vi "Plugin Page.vi"(8 "error in (no error)":errorcluster, 11 "Node Ptr":T1 format="%.0x") -> (0 "error out":errorcluster)   [LabVIEW 2020, in "DSF System Explorer.lvlib"]
uses:
  DSF System Explorer.lvlib
  <vilib>/NI VeriStand/Custom Device API/Custom Device Item Ref.ctl
  DSF Core.lvlibp/Classes/Component User Interface/UI Type.ctl
  <vilib>/NI VeriStand/Custom Device API/Custom Device API.lvlib
  DSF Shared.lvlib
  DSF Core.lvlibp/Classes/Component User Interface/Component User Interfaces.lvclass
  DSF Core.lvlibp/Classes/User Interface/User Interface.lvclass
panel:
  in  "Tab Control":enum32{"Settings"}(tab)
  in  "Priority":u64
  in  "Decimation":u64
  in  "Offset":u64
  in  "Header":cluster{"Section Name":string}={"Section Name"="Plugin"}
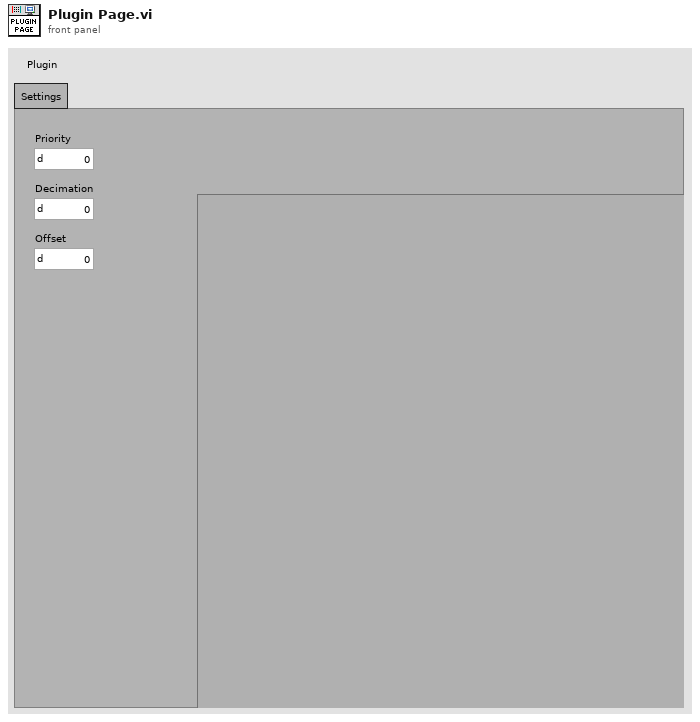
[diagram p1: front panel]
types:
  T1 = typedef "Custom Device API.lvlib/Custom Device Item Ref.ctl" = u64
  T2 = typedef "DSF Core.lvlibp/Component User Interfaces.lvclass/UI Type.ctl" = enum16{"Plugin", "Thread", "Rx Group", "Tx Group", "Rx Transfer", "Tx Transfer", "Rx Channel", "Tx Channel"}
  T3 = typedef "DSF Core.lvlibp/Plugin Configuration.lvclass/Core Plugin Configuration.ctl" = cluster{"name":string, "components":string[], "cycle timing":T4}
  T4 = typedef "DSF Core.lvlibp/DSF Timing Info.ctl" = cluster{"priority":u64, "decimation":u64, "offset":u64}
  T5 = typedef "DSF Core.lvlibp/User Interface Handler.lvclass/User Interface Ref.ctl" = refnum<vi>
  T6 = typedef "DSF Core.lvlibp/DSF Settings Info.ctl" = cluster{"component":string, "values":cluster{"key":string, "value":string}[]}
  T7 = typedef "Custom Device API.lvlib/Custom Device Commands.ctl" = enum16{"Default", "Item renamed", "Shutdown", "Dynamic button pressed"}
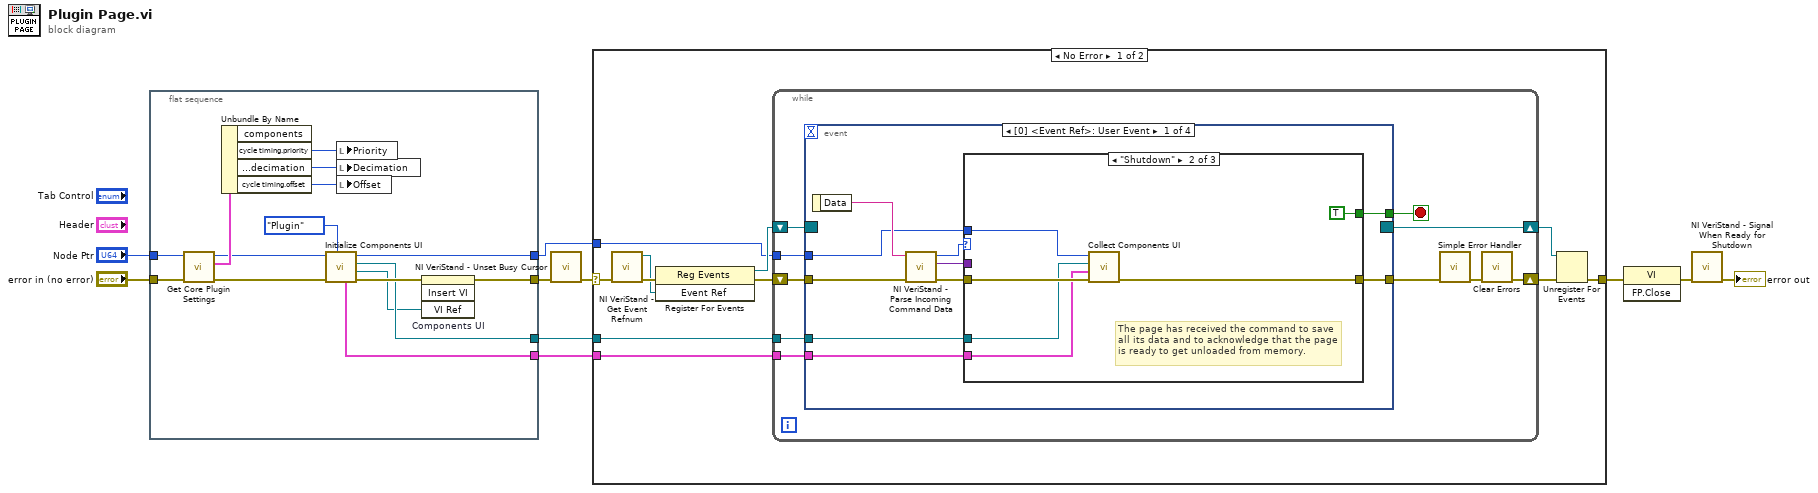
[diagram p0: block diagram]
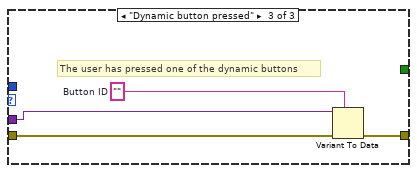
[diagram p3: hidden frame]
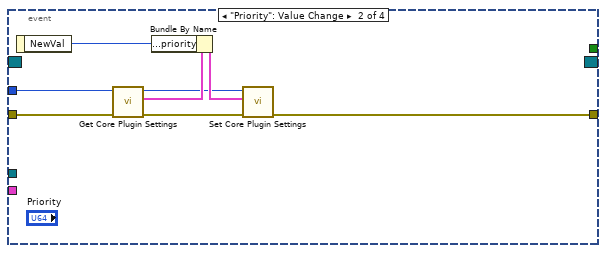
[diagram p4: hidden frame]
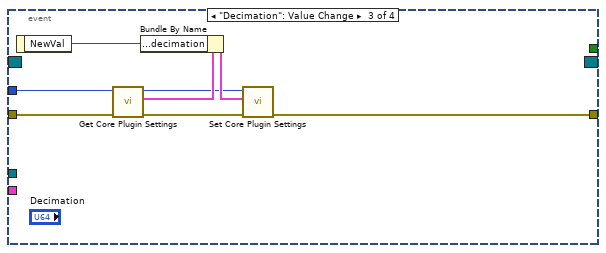
[diagram p5: hidden frame]
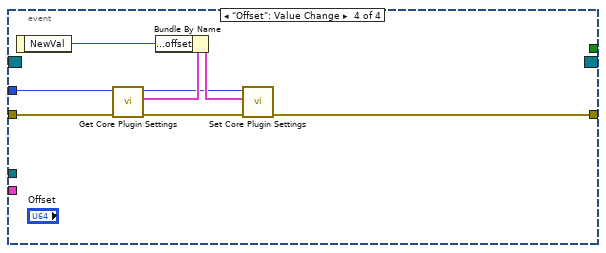
[diagram p6: hidden frame]
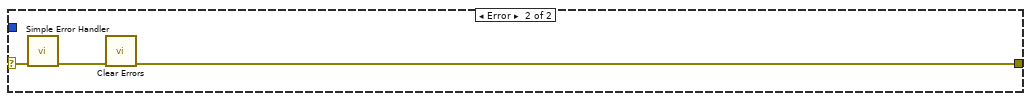
[diagram p7: hidden frame]
diagram:
  n1 = flat-sequence "Initialization code" {
    tunnel: "error in (no error)" -> [w24]
    tunnel: "Node Ptr" -> [w23]
    tunnel: [w11] -> w6
    tunnel: [w16] -> w3
    tunnel: [w15] -> w2
    tunnel: [w12] -> w1
    frame #0 {
      n2 = call "Get Core Plugin Settings.vi"("error in (no error)"=w24, "Item Ref in"=w23) -> ("error out"=w18:errorcluster, "plugin configuration"=w19:T3, "Item Ref out"=w17:T1)  [unwired: 7 in]
      n3 = Unbundle By Name(w19) -> ("cycle timing.priority"=w20:u64, "cycle timing.decimation"=w22:u64, "cycle timing.offset"=w21:u64)  [unwired: 1 out]
      n4 = call "Initialize Components UI.vi"("user interface type"=UI_Type."Plugin", "error in (no error)"=w18, "Item Ref in"=w17) -> ("error out"=w25:errorcluster, "active vi"=w14:T5, "User Interface Handler"=w15:refnum<class "User Interface Handler.lvclass">, "Item Ref out"=w16:T1, "component settings"=w12:T6[])  [unwired: 4 in]
      n5 = local write "Priority"(w20) -> ()
      n6 = local write "Decimation"(w22) -> ()
      n7 = local write "Offset"(w21) -> ()
      n8 = invoke on="Components UI" class="SubPnl" method="Insert VI"(error in=w25, "VI Ref"=w14) -> (error out=w11:errorcluster)  [unwired: 2 in, 3 out]
    }
  }
  n9 = call <vilib>:"NI VeriStand - Unset Busy Cursor.vi"("error in (no error)"=w6) -> ("error out"=w5:errorcluster)  [unwired: 10 out]
  n10 = case shown="No Error" w5 {
    selector: w5 -> [w28 w94]
    tunnel: [w33 w92] -> w10
    tunnel: w3 -> [w29 _]
    tunnel: w2 -> [w27 _]
    tunnel: w1 -> [w26 _]
    frame No Error {
      n11 = call <vilib>:"NI VeriStand - Get Event Refnum.vi"("error in (no error)"=w28) -> ("error out"=w36:errorcluster, "Event Ref"=w32:refnum<user-event>)  [unwired: 9 out]
      n12 = register-events(error in=w36, w32) -> (reference out=w30:refnum<event-registration>, error out=w31:errorcluster)  [unwired: 1 in]
      n13 = while {
        tunnel: w29 -> [w42]
        shift-right: [w39] -> w34
        shift-left: w31 -> [w45]
        shift-right: [w46] -> w35
        shift-left: w30 -> [w44]
        tunnel: w27 -> [w38]
        tunnel: w26 -> [w37]
        stop <- w43 stop-if-true
        n14 = event shown="[0] <Event Ref>: User Event" {
          selector: w44 -> [_ _ _ _]
          dyn-events: [_ _ _ _] -> w46
          timeout: _ -> [_ _ _ _]
          tunnel: w45 -> [w56 w75 w83 w91]
          tunnel: [w52 _ _ _] -> w43
          tunnel: [w51 w68 w76 w84] -> w41
          tunnel: w42 -> [w50 w74 w82 w90]
          tunnel: w38 -> [w48 _ _ _]
          tunnel: w37 -> [w47 _ _ _]
          event User Event {
            n15 = event-data() -> ("Data"=w55:string)  [unwired: 1 out]
            n16 = call <vilib>:"NI VeriStand - Parse Incoming Command Data.vi"("error in (no error)"=w56, "Incoming data"=w55) -> ("error out"=w54:errorcluster, "Outgoing data"=w49:variant, "Action"=w53:T7)  [unwired: 7 out]
            n17 = case shown="\"Shutdown\"" w53 {
              tunnel: w54 -> [w57 w62 w67]
              tunnel: [_ TRUE _] -> w52
              tunnel: [w57 w61 w64] -> w51
              tunnel: w50 -> [_ w59 _]
              tunnel: w49 -> [_ _ w66]
              tunnel: w48 -> [_ w60 _]
              tunnel: w47 -> [_ w58 _]
              frame "Default", Default {
              }
              frame "Shutdown" {
                # "The page has received the command to save all its data and to acknowledge that the page is ready to get unloaded from memory."
                n18 = call "Collect Components UI.vi"("error in (no error)"=w62, "current component settings"=w58, "User Interface Handler"=w60, "Item Ref in"=w59) -> ("error out"=w61:errorcluster)  [unwired: 6 in, 1 out]
              }
              frame "Dynamic button pressed" {
                w65 = ""  # Button ID
                # "The user has pressed one of the dynamic buttons"
                n19 = Variant To Data(error in=w67, type=w65, Variant=w66) -> (error out=w64:errorcluster)  [unwired: 1 out]
              }
            }
          }
          event "Priority": Value Change {
            n20 = event-data() -> ("NewVal"=w73:u64)  [unwired: 1 out]
            n21 = call "Get Core Plugin Settings.vi"("error in (no error)"=w75, "Item Ref in"=w74) -> ("error out"=w71:errorcluster, "plugin configuration"=w72:T3, "Item Ref out"=w69:T1)  [unwired: 7 in]
            n22 = Bundle By Name(cluster=w72, "cycle timing.priority"=w73) -> (w70:T3)
            n23 = call "Set Core Plugin Settings.vi"("error in (no error)"=w71, "plugin configuration"=w70, "Item Ref in"=w69) -> ("error out"=w68:errorcluster)  [unwired: 7 in, 1 out]
          }
          event "Decimation": Value Change {
            n24 = event-data() -> ("NewVal"=w81:u64)  [unwired: 1 out]
            n25 = call "Get Core Plugin Settings.vi"("error in (no error)"=w83, "Item Ref in"=w82) -> ("error out"=w79:errorcluster, "plugin configuration"=w80:T3, "Item Ref out"=w77:T1)  [unwired: 7 in]
            n26 = Bundle By Name(cluster=w80, "cycle timing.decimation"=w81) -> (w78:T3)
            n27 = call "Set Core Plugin Settings.vi"("error in (no error)"=w79, "plugin configuration"=w78, "Item Ref in"=w77) -> ("error out"=w76:errorcluster)  [unwired: 7 in, 1 out]
          }
          event "Offset": Value Change {
            n28 = event-data() -> ("NewVal"=w89:u64)  [unwired: 1 out]
            n29 = call "Get Core Plugin Settings.vi"("error in (no error)"=w91, "Item Ref in"=w90) -> ("error out"=w87:errorcluster, "plugin configuration"=w88:T3, "Item Ref out"=w85:T1)  [unwired: 7 in]
            n30 = Bundle By Name(cluster=w88, "cycle timing.offset"=w89) -> (w86:T3)
            n31 = call "Set Core Plugin Settings.vi"("error in (no error)"=w87, "plugin configuration"=w86, "Item Ref in"=w85) -> ("error out"=w84:errorcluster)  [unwired: 7 in, 1 out]
          }
        }
        n32 = call <vilib>:"Simple Error Handler.vi"("error in (no error)"=w41) -> ("error out"=w40:errorcluster)  [unwired: 1 in, 7 out]
        n33 = call <vilib>:"Clear Errors.vi"("error in (no error)"=w40) -> ("error out"=w39:errorcluster)  [unwired: 1 in, 5 out]
      }
      n34 = Unregister For Events(event registration refnum=w35, error in=w34) -> (error out=w33:errorcluster)
    }
    frame Error {
      n35 = call <vilib>:"Simple Error Handler.vi"("error in (no error)"=w94) -> ("error out"=w93:errorcluster)  [unwired: 1 in, 7 out]
      n36 = call <vilib>:"Clear Errors.vi"("error in (no error)"=w93) -> ("error out"=w92:errorcluster)  [unwired: 1 in, 5 out]
    }
  }
  n37 = invoke class="VI" method="FP.Close"(error in=w10) -> (error out=w9:errorcluster)  [unwired: 2 in, 2 out]
  n38 = call <vilib>:"NI VeriStand - Signal When Ready for Shutdown.vi"("error in (no error)"=w9) -> ("error out"=→"error out":errorcluster)  [unwired: 10 out]
